vi "ModelPath.vi"() -> (0 "error out":errorcluster, 1 "found?":bool, 2 "Models":string[](array[string]), 3 "Refnum out":T1)   [LabVIEW 2013]
uses:
  <vilib>/Utility/config.llb/Config Data RefNum.ctl
  <vilib>/Utility/config.llb/Read Key (String).vi
  <vilib>/Utility/config.llb/NI_LVConfig.lvlib
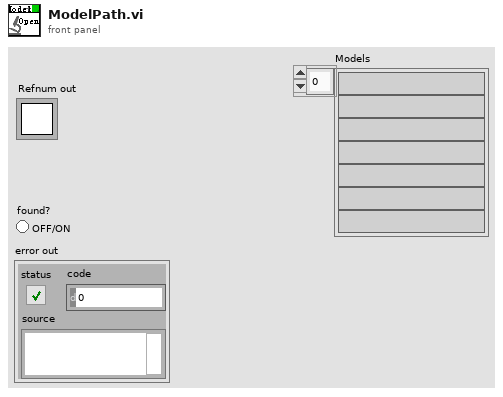
[diagram p1: front panel]
types:
  T1 = typedef "NI_LVConfig.lvlib/Config Data RefNum.ctl" = refnum<k1>
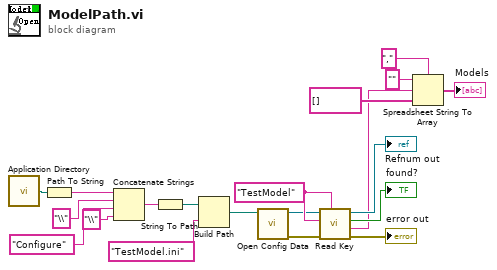
[diagram p0: block diagram]
diagram:
  w9 = "TestModel" ("section")
  n1 = call <vilib>:"Application Directory.vi"() -> ("Application Directory"=w12:path)
  n2 = Path To String(path=w12) -> (string=w13:string)
  n3 = Concatenate Strings(w13, "\\" ("string"), "Configure" ("string"), "\\" ("string")) -> (w16:string)
  n4 = String To Path(string=w16) -> (path=w18:path)
  n5 = Build Path(base path=w18, name or relative path="TestModel.ini") -> (appended path=w10:path)
  n6 = call <vilib>:"Open Config Data.vi"("configuration file path"=w10) -> ("error out"=w7:errorcluster, "refnum"=w8:T1)  [unwired: 8 in, 1 out]
  n7 = call-poly <vilib>:"Read Key.vi"("section"=w9, "error in (no error)"=w7, "key"=w9, "refnum"=w8) -> ("error out"=→"error out":errorcluster, "value"=w2:string, "found?"=→"found?":bool, "refnum out"=→"Refnum out":T1)  [unwired: 4 in]
  n8 = Spreadsheet String To Array(delimiter (Tab)=",", format string="", spreadsheet string=w2, array type (2D Dbl)=string[] []) -> (array=→"Models":string[])
